vi "Logger_Init.vi"(0 "object in":refnum<class "Logger.lvclass">, 2 "LogString":refnum<vi>, 5 "error in (no error)":errorcluster) -> (14 "object out":refnum<class "Logger.lvclass">, 19 "error out":errorcluster)   [LabVIEW 2014, in "Logger.lvclass"]
uses:
  Logger.lvclass
  Logger.lvclass/Logger.ctl
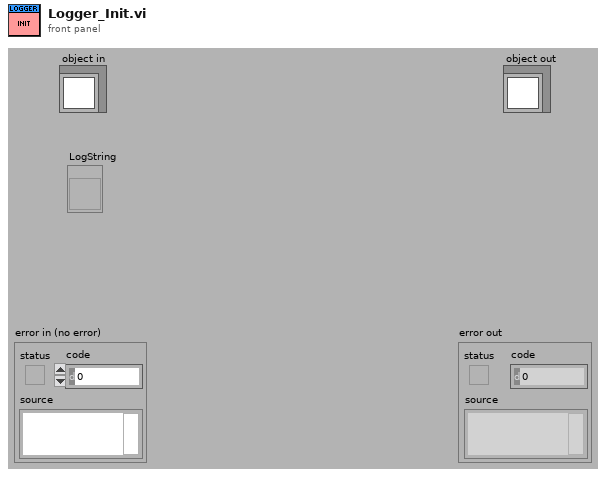
[diagram p1: front panel]
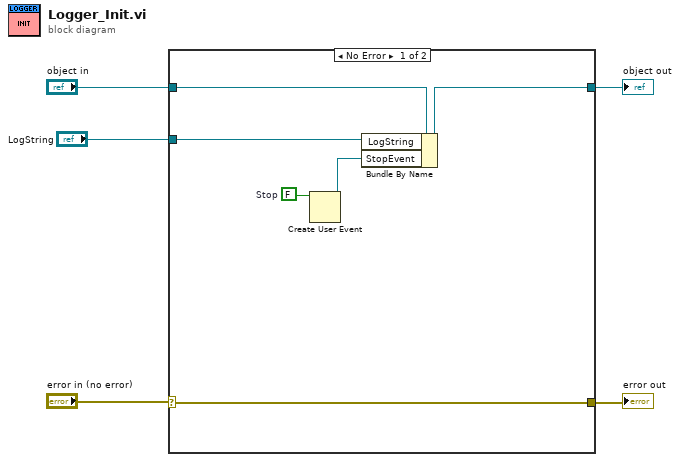
[diagram p0: block diagram]
diagram:
  n1 = case shown="No Error" "error in (no error)" {
    selector: "error in (no error)" -> [w9 w12]
    tunnel: "object in" -> [w11 w13]
    tunnel: [w10 w13] -> w4
    tunnel: [w9 w12] -> w2
    tunnel: "LogString" -> [w8 _]
    frame No Error {
      w6 = FALSE  # Stop
      n2 = Create User Event(user event datatype=w6) -> (user event=w7:refnum<user-event>)  [unwired: 1 in, 1 out]
      n3 = Bundle By Name(cluster=w11, "LogString"=w8, "StopEvent"=w7) -> (w10:refnum<class "Logger.lvclass">)
    }
    frame Error {
    }
  }
  "object out" <- w4
  "error out" <- w2
